vi "WRO_moTEST.vi"() -> ()   [LabVIEW 2014]
uses:
  <vilib>/myRIO/Instrument Drivers/Onboard IO/AI/vis/Read.vi
  <vilib>/myRIO/Instrument Drivers/Onboard IO/AI/vis/Smart Open.vi
  <vilib>/Utility/error.llb/Error Cluster From Error Code.vi
  <vilib>/myRIO/Common/Instrument Driver Framework/myRIO v1.0/AI/vis/myRIO v1.0 Read AI.vi
panel:
  out "2":dbl=-0.0634765559999999
  out "1":dbl=-0.0402831990000001
  out "0":dbl=-0.015869138999999866
  out "웨이브폼 차트":dbl[](graph)=[2.7978512760000003, 2.8527829110000003, 2.8955075160000003]
  out "Col02 (B/AI2 (Pin 7))":dbl=2.8955075160000003
  out "Col01 (B/AI1 (Pin 5))":dbl=2.8527829110000003
  out "Col00 (B/AI0 (Pin 3))":dbl=2.7978512760000003
  in  "불리언 6":bool=TRUE
  in  "불리언 5":bool=TRUE
  in  "불리언 4":bool=TRUE
  in  "불리언 3":bool
  in  "불리언 2":bool=TRUE
  in  "불리언":bool=TRUE
  in  "3_1M":i32
  in  "3_2M":i32
  in  "2_2M":i32
  in  "2_1M":i32
  in  "subM_6":u8(slide)=125 step=1 scale=0.0..255.0
  in  "subM_5":u8(slide)=120 step=1 scale=0.0..255.0
  in  "subM_4":u8(slide)=122 step=1 scale=0.0..255.0
  in  "subM_3":u8(slide)=128 step=1 scale=0.0..255.0
  in  "subM_2":u8(slide)=230 step=1 scale=0.0..255.0
  in  "subM_1":u8(slide)=128 step=1 scale=0.0..255.0
  in  "정지":bool
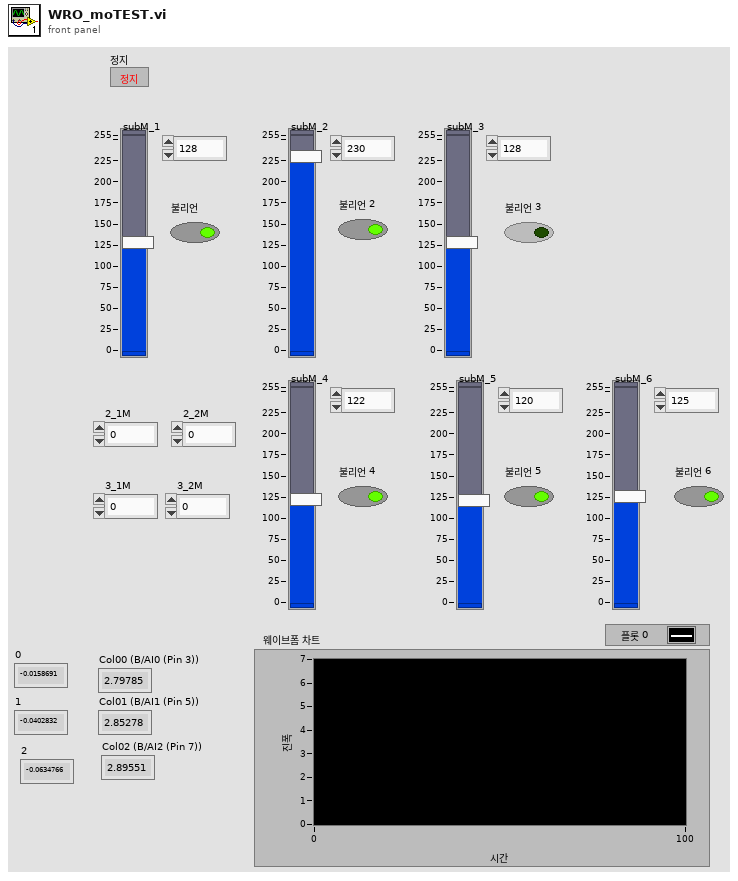
[diagram p1: front panel]
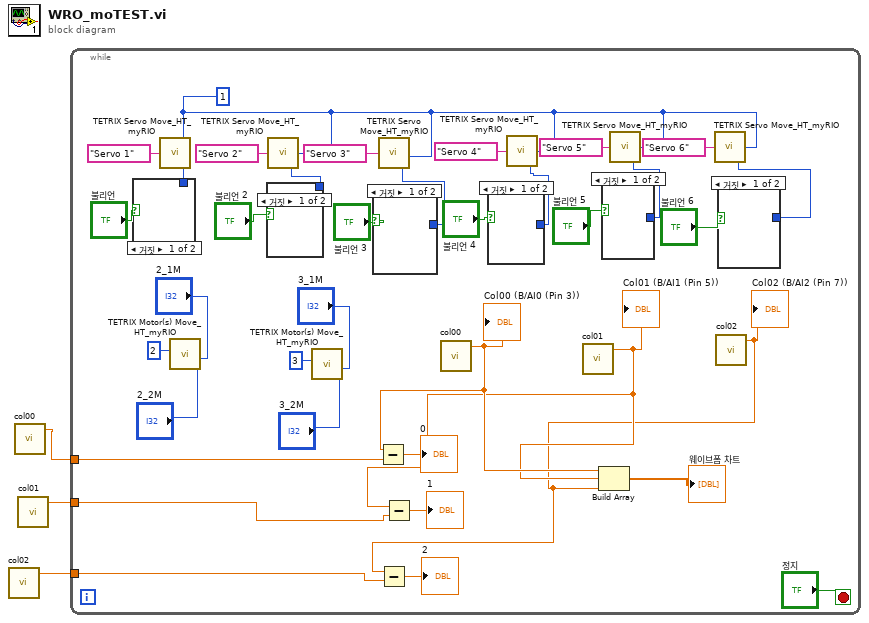
[diagram p0: block diagram]
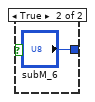
[diagram p2: hidden frame]
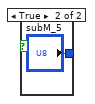
[diagram p3: hidden frame]
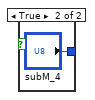
[diagram p4: hidden frame]
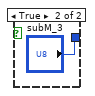
[diagram p5: hidden frame]
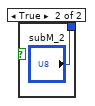
[diagram p6: hidden frame]
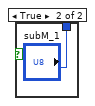
[diagram p7: hidden frame]
diagram:
  n1 = call "col02.vi"() -> ("Col02 (B/AI2 (Pin 7))"=w1:dbl)  [unwired: 26 in, 1 out]
  n2 = call "col00.vi"() -> ("Col00 (B/AI0 (Pin 3))"=w3:dbl)  [unwired: 26 in, 1 out]
  n3 = call "col01.vi"() -> ("Col01 (B/AI1 (Pin 5))"=w2:dbl)  [unwired: 26 in, 1 out]
  n4 = while {
    tunnel: w3 -> [w9]
    tunnel: w2 -> [w8]
    tunnel: w1 -> [w7]
    stop <- "정지" stop-if-true
    w38 = u8 1 ("Controller Daisy Chain Position (1 - 4)")
    n5 = case shown="거짓" "불리언" {
      tunnel: [_ "subM_1"] -> w24
      frame False {
      }
      frame True {
      }
    }
    n6 = call <vilib>:"TETRIX Servo Move_HT_myRIO.vi"("Servo Position (0 - 255)"=w24, "Controller Daisy Chain Position (1 - 4)"=w38, "Select Servo"="Servo 1") -> ()  [unwired: 2 in, 1 out]
    n7 = call <vilib>:"TETRIX Motor(s) Move_HT_myRIO.vi"("Motor 2 Power (-100 to 100)\n0 = Stop/Brake\n-128 = Stop/Coast"="2_2M", "Motor 1 Power (-100 to 100)\n0 = Stop/Brake\n-128 = Stop/Coast"="2_1M", "Controller Daisy Chain Position: 1 - 4"=u8 2) -> ()  [unwired: 6 in, 1 out]
    n8 = case shown="거짓" "불리언 2" {
      tunnel: [_ "subM_2"] -> w18
      frame False {
      }
      frame True {
      }
    }
    n9 = call <vilib>:"TETRIX Servo Move_HT_myRIO.vi"("Servo Position (0 - 255)"=w18, "Controller Daisy Chain Position (1 - 4)"=w38, "Select Servo"="Servo 2") -> ()  [unwired: 2 in, 1 out]
    n10 = call <vilib>:"TETRIX Motor(s) Move_HT_myRIO.vi"("Motor 2 Power (-100 to 100)\n0 = Stop/Brake\n-128 = Stop/Coast"="3_2M", "Motor 1 Power (-100 to 100)\n0 = Stop/Brake\n-128 = Stop/Coast"="3_1M", "Controller Daisy Chain Position: 1 - 4"=u8 3) -> ()  [unwired: 6 in, 1 out]
    n11 = case shown="거짓" "불리언 3" {
      tunnel: [_ "subM_3"] -> w17
      frame False {
      }
      frame True {
      }
    }
    n12 = call <vilib>:"TETRIX Servo Move_HT_myRIO.vi"("Servo Position (0 - 255)"=w17, "Controller Daisy Chain Position (1 - 4)"=w38, "Select Servo"="Servo 3") -> ()  [unwired: 2 in, 1 out]
    n13 = call "col00.vi"() -> ("Col00 (B/AI0 (Pin 3))"=w12:dbl)  [unwired: 26 in, 1 out]
    "Col00 (B/AI0 (Pin 3))" <- w12
    n14 = Subtract(x=w12, y=w9) -> (x-y=→"0":dbl)
    n15 = case shown="거짓" "불리언 4" {
      tunnel: [_ "subM_4"] -> w16
      frame False {
      }
      frame True {
      }
    }
    n16 = call <vilib>:"TETRIX Servo Move_HT_myRIO.vi"("Servo Position (0 - 255)"=w16, "Controller Daisy Chain Position (1 - 4)"=w38, "Select Servo"="Servo 4") -> ()  [unwired: 2 in, 1 out]
    n17 = call "col01.vi"() -> ("Col01 (B/AI1 (Pin 5))"=w11:dbl)  [unwired: 26 in, 1 out]
    "Col01 (B/AI1 (Pin 5))" <- w11
    n18 = Subtract(x=w11, y=w8) -> (x-y=→"1":dbl)
    n19 = case shown="거짓" "불리언 5" {
      tunnel: [_ "subM_5"] -> w15
      frame False {
      }
      frame True {
      }
    }
    n20 = call <vilib>:"TETRIX Servo Move_HT_myRIO.vi"("Servo Position (0 - 255)"=w15, "Controller Daisy Chain Position (1 - 4)"=w38, "Select Servo"="Servo 5") -> ()  [unwired: 2 in, 1 out]
    n21 = call "col02.vi"() -> ("Col02 (B/AI2 (Pin 7))"=w10:dbl)  [unwired: 26 in, 1 out]
    "Col02 (B/AI2 (Pin 7))" <- w10
    n22 = Subtract(x=w10, y=w7) -> (x-y=→"2":dbl)
    n23 = Build Array(w12, w11, w10) -> (→"웨이브폼 차트":dbl[])
    n24 = case shown="거짓" "불리언 6" {
      tunnel: [_ "subM_6"] -> w14
      frame False {
      }
      frame True {
      }
    }
    n25 = call <vilib>:"TETRIX Servo Move_HT_myRIO.vi"("Servo Position (0 - 255)"=w14, "Controller Daisy Chain Position (1 - 4)"=w38, "Select Servo"="Servo 6") -> ()  [unwired: 2 in, 1 out]
  }
